vi "Ramp 전압.vi"() -> ()   [LabVIEW 2019]
panel:
  out "Waveform Chart":dbl(graph)
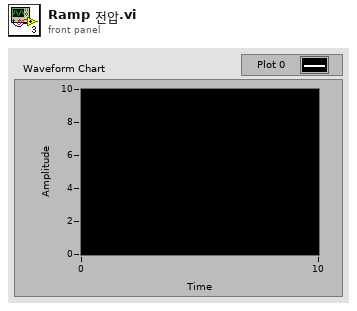
[diagram p1: front panel]
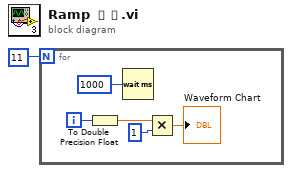
[diagram p0: block diagram]
diagram:
  n1 = for {
    N: 11 -> [_]
    i -> [w4]
    n2 = To Double Precision Float(number=w4) -> (double precision float=w5:dbl)
    n3 = Wait (ms)(milliseconds to wait=1000) -> ()  [unwired: 1 out]
    n4 = Multiply(x=w5, y=1) -> (x*y=→"Waveform Chart":dbl)
  }
